vi "initialize timing source.vi"(8 "error in":errorcluster, 11 "timing source in":refnum<class "TBM timing source.lvclass">) -> (0 "error out":errorcluster, 3 "timing source out":refnum<class "TBM timing source.lvclass">)   [LabVIEW 2013, in "TBM timing source.lvclass"]
doc: "An interface for initializing a timing source. In many cases this may be a no-op. There is no expectation about when this function should be called, but it must be called before entering the loop to be timed."
uses:
  TBM timing source.lvclass
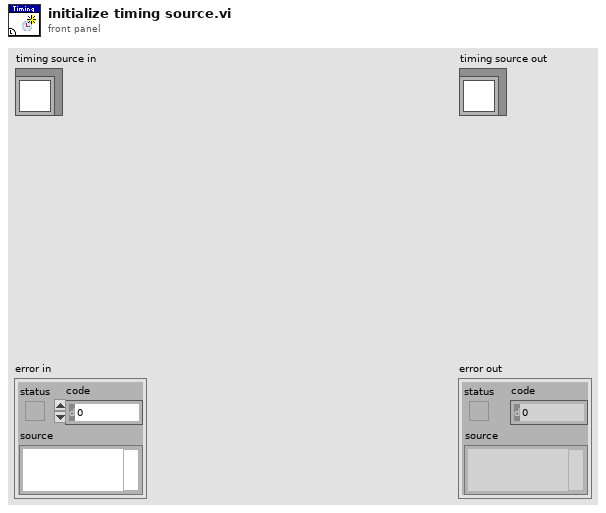
[diagram p1: front panel]
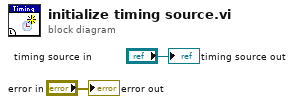
[diagram p0: block diagram]
diagram:
  "error out" <- "error in"
  "timing source out" <- "timing source in"
